vi "S2DS_ConfigWriteRC (SubVI).vi"(0 "Refnum in":T1, 1 "RC info list":T2, 3 "error in":errorcluster) -> (6 "Refnum out":T1, 9 "error out":errorcluster)   [LabVIEW 2025]
uses:
  <vilib>/Utility/config.llb/Config Data RefNum.ctl
  TYPE DEFS/S2DS_RC info.ctl
  TYPE DEFS/S2DS_Single RC info.ctl
  <vilib>/Utility/config.llb/Write Key (U32).vi
  <vilib>/Utility/config.llb/Write Key (String).vi
  <vilib>/Utility/config.llb/Write Key (Double).vi
  <vilib>/Utility/config.llb/Write Key (I32).vi
  <vilib>/Utility/config.llb/NI_LVConfig.lvlib
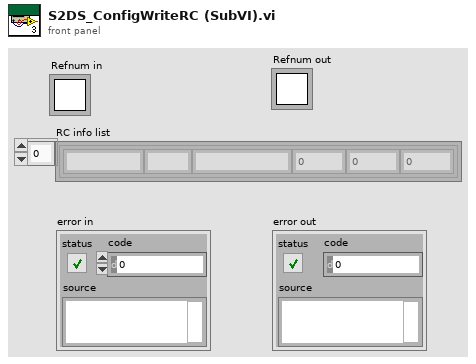
[diagram p1: front panel]
types:
  T1 = typedef "NI_LVConfig.lvlib/Config Data RefNum.ctl" = refnum<k1>
  T2 = typedef "S2DS_RC info.ctl" = T3[]
  T3 = typedef "S2DS_Single RC info.ctl" = cluster{"Instrument identifier":string, "Factor":dbl, "Averaging":i32, "Wait (ms)":i32, "Unit":string, "Name":string}
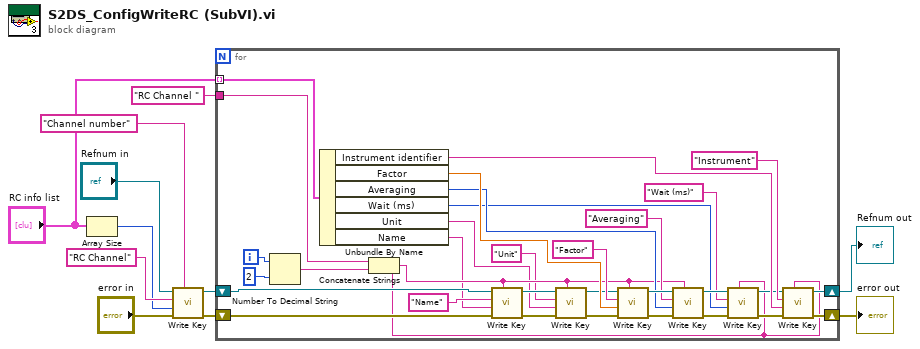
[diagram p0: block diagram]
diagram:
  n1 = Array Size(array="RC info list") -> (size(s)=w1:i32)
  n2 = call-poly <vilib>:"Write Key.vi"("section"="Channel number", "error in (no error)"="error in", "value"=w1, "key"="RC Channel", "refnum"="Refnum in") -> ("error out"=w3:errorcluster, "refnum out"=w4:T1)  [unwired: 4 in, 1 out]
  n3 = for {
    tunnel: "RC info list" -> [w43] mode=indexing
    tunnel: "RC Channel " -> [w38]
    shift-right: [w18] -> w11
    shift-left: w3 -> [w22]
    shift-right: [w17] -> w9
    shift-left: w4 -> [w21]
    i -> [w40]
    n4 = Number To Decimal String(number=w40, width (-)=i16 2) -> (decimal integer string=w37:string)
    n5 = Unbundle By Name(w43) -> ("Instrument identifier"=w36:string, "Factor"=w35:dbl, "Averaging"=w34:i32, "Wait (ms)"=w33:i32, "Unit"=w13:string, "Name"=w12:string)
    n6 = Concatenate Strings(w38, w37) -> (w16:string)
    n7 = call-poly <vilib>:"Write Key.vi"("section"=w16, "error in (no error)"=w22, "value"=w12, "key"="Name", "refnum"=w21) -> ("error out"=w24:errorcluster, "refnum out"=w26:T1)  [unwired: 4 in, 1 out]
    n8 = call-poly <vilib>:"Write Key.vi"("section"=w16, "error in (no error)"=w24, "value"=w13, "key"="Unit", "refnum"=w26) -> ("error out"=w23:errorcluster, "refnum out"=w25:T1)  [unwired: 4 in, 1 out]
    n9 = call-poly <vilib>:"Write Key.vi"("section"=w16, "error in (no error)"=w23, "value"=w35, "key"="Factor", "refnum"=w25) -> ("error out"=w32:errorcluster, "refnum out"=w42:T1)  [unwired: 4 in, 1 out]
    n10 = call-poly <vilib>:"Write Key.vi"("section"=w16, "error in (no error)"=w32, "value"=w34, "key"="Averaging", "refnum"=w42) -> ("error out"=w31:errorcluster, "refnum out"=w41:T1)  [unwired: 4 in, 1 out]
    n11 = call-poly <vilib>:"Write Key.vi"("section"=w16, "error in (no error)"=w31, "value"=w33, "key"="Wait (ms)", "refnum"=w41) -> ("error out"=w19:errorcluster, "refnum out"=w20:T1)  [unwired: 4 in, 1 out]
    n12 = call-poly <vilib>:"Write Key.vi"("section"=w16, "error in (no error)"=w19, "value"=w36, "key"="Instrument", "refnum"=w20) -> ("error out"=w18:errorcluster, "refnum out"=w17:T1)  [unwired: 4 in, 1 out]
  }
  "error out" <- w11
  "Refnum out" <- w9
